vi "AeroFlowSanitiser.vi"(9 "Error_Flags":dbl[](array[numeric])=[200000.0, 200000.0, 200000.0, 200000.0, 200001.0, 200000.0, 200001.0, 200000.0, 200001.0, 200000.0, 200000.0, 200000.0, 200000.0, 200001.0, 200000.0, 200001.0, 200000.0, 200001.0, 200000.0, 200000.0, 200001.0, 200001.0, 200001.0, 200000.0, 200001.0, 200000.0, 200001.0, 200000.0, 200001.0, 200001.0, 200000.0, 200001.0, 200001.0, 200001.0, 200000.0, 200001.0, 200000.0, 200000.0, 200000.0, 200001.0, 200001.0, 200001.0, 200000.0, 200000.0, 200000.0, 200000.0, 200000.0, 200000.0, 200001.0, 200000.0, 200001.0, 200001.0, 200001.0, 200000.0, 200001.0, 200000.0, 200000.0, 200000.0, 200000.0, 200001.0, 200000.0, 200001.0, 200000.0, 200001.0, 200001.0, 200001.0, 200001.0, 200001.0, 200001.0, 200001.0, 200001.0, 200001.0, 200001.0, 200001.0, 200001.0, 200001.0, 200001.0, 200001.0, 200000.0, 200001.0, 200001.0, 200001.0, 200001.0, 200001.0, 200000.0, 200000.0, 200001.0, 200000.0, 200000.0, 200000.0, 200001.0, 200001.0, 200000.0, 200001.0, 200000.0, 200000.0, 200000.0, 200000.0, 200000.0, 200000.0, 200000.0, 200001.0, 200000.0, 200001.0, 200000.0, 200000.0, 200000.0, 200000.0, 200000.0, 200000.0, 200000.0, 200000.0, 200000.0, 200000.0, 200000.0, 200001.0, 200001.0, 200001.0, 200000.0, 200000.0, 200000.0, 200000.0, 200001.0, 200000.0, 200000.0, 200000.0, 200001.0, 200001.0, 200000.0, 200000.0, 200000.0, 200001.0, 200000.0, 200000.0, 200001.0, 200000.0, 200001.0, 200001.0, 200001.0, 200000.0, 200001.0, 200001.0, 200001.0, 200001.0, 200001.0, 200001.0, 200001.0, 200001.0, 200001.0, 200001.0, 200001.0, 200001.0, 200001.0, 200000.0, 200000.0, 200000.0, 200000.0, 200000.0, 200001.0, 200001.0, 200001.0, 200001.0, 200001.0, 200001.0, 200001.0, 200001.0, 200001.0, 200001.0, 200001.0, 200000.0, 200001.0, 200001.0, 200001.0, 200001.0, 200001.0, 200001.0, 200000.0, 200001.0, 200001.0, 200001.0, 200001.0, 200001.0, 200001.0, 200000.0, 200001.0, 200001.0, 200001.0, 200000.0, 200001.0, 200000.0, 200000.0, 200001.0, 200001.0, 200001.0, 200001.0, 200001.0, 200001.0, 200000.0, 200000.0, 200000.0, 200001.0, 200001.0, 200001.0, 200001.0, 200000.0, 200001.0, 200001.0, 200001.0, 200001.0, 200000.0, 200001.0, 200001.0, 200001.0, 200001.0, 200000.0, 200001.0, 200000.0, 200001.0, 200001.0, 200001.0, 200001.0, 200001.0, 200001.0, 200001.0, 200001.0, 200001.0, 200001.0, 200001.0, 200001.0, 200001.0, 200001.0, 200001.0, 200001.0, 200001.0, 200000.0, 200001.0, 200001.0, 200001.0, 200001.0, 200001.0, 200000.0, 200001.0, 200001.0, 200001.0, 200000.0, 200000.0, 200001.0, 200000.0, 200001.0, 200001.0, 200001.0, 200001.0, 200001.0, 200001.0, 200001.0, 200001.0, 200001.0, 200001.0, 200001.0, 200001.0, 200000.0, 200001.0, 200001.0, 200000.0, 200001.0, 200000.0, 200001.0, 200000.0, 200001.0, 200001.0, 200001.0, 200001.0, 200001.0, 200001.0, 200001.0, 200000.0, 200001.0, 200001.0, 200000.0, 200001.0, 200001.0, 200001.0, 200001.0, 200001.0, 200000.0, 200001.0, 200001.0, 200001.0, 200000.0, 200001.0, 200000.0, 200000.0, 200001.0, 200001.0, 200001.0, 200000.0, 200001.0, 200000.0, 200001.0, 200000.0, 200000.0, 200000.0, 200000.0, 200000.0, 200000.0, 200001.0, 200000.0, 200000.0, 200000.0, 200000.0, 200000.0, 200001.0, 200000.0, 200000.0, 200001.0, 200001.0, 200001.0, 200000.0, 200000.0, 200100.0, 200000.0, 200001.0, 200001.0, 200001.0, 200000.0, 200001.0, 200001.0, 200001.0, 200000.0, 200001.0, 200000.0, 200001.0, 200000.0, 200000.0, 200000.0, 200000.0, 200000.0, 200000.0, 200000.0, 200000.0, 200001.0, 200001.0, 200001.0, 200001.0, 200000.0, 200001.0, 200001.0, 200001.0, 200001.0, 200001.0, 200001.0, 200001.0, 200001.0, 200001.0, 200001.0, 200001.0, 200001.0, 200001.0, 200000.0, 200000.0, 200001.0, 200000.0, 200000.0, 200001.0, 200001.0, 200001.0, 200000.0, 200001.0, 200000.0, 200000.0, 200001.0, 200000.0, 200000.0, 200001.0, 200001.0, 200000.0, 200001.0, 200001.0, 200100.0, 200001.0, 200001.0, 200001.0, 200001.0, 200000.0, 200001.0, 200000.0, 200001.0, 200001.0, 200001.0, 200001.0, 200001.0, 200001.0, 200000.0, 200001.0, 200000.0, 200001.0, 200001.0, 200001.0, 200000.0, 200001.0, 200000.0, 200001.0, 200000.0, 200000.0, 200001.0, 200001.0, 200001.0, 200001.0, 200001.0, 200001.0, 200000.0, 200000.0, 200001.0, 200001.0, 200001.0, 200001.0, 200000.0, 200001.0, 200000.0, 200001.0, 200001.0, 200001.0, 200001.0, 200001.0, 200001.0, 200001.0, 200001.0, 200001.0, 200001.0, 200001.0, 200001.0, 200001.0, 200001.0, 200001.0, 200001.0, 200001.0, 200000.0, 200000.0, 200000.0, 200000.0, 200000.0, 200000.0, 200001.0, 200001.0, 200000.0, 200001.0, 200000.0, 200001.0, 200001.0, 200001.0, 200000.0, 200001.0, 200000.0, 200001.0, 200001.0, 200000.0, 200001.0, 200000.0, 200001.0, 200001.0, 200000.0, 200100.0, 200001.0, 200001.0, 200000.0, 200001.0, 200001.0, 200001.0, 200001.0, 200001.0, 200001.0, 200001.0, 200000.0, 200001.0, 200000.0, 200000.0, 200001.0, 200001.0, 200001.0, 200001.0, 200001.0, 200001.0, 200001.0, 200001.0, 200001.0, 200001.0, 200001.0, 200001.0, 200001.0, 200001.0, 200001.0, 200001.0, 200001.0, 200100.0, 200000.0, 200001.0, 200001.0, 200001.0, 200001.0, 200000.0, 200001.0, 200001.0, 200001.0, 200000.0, 200001.0, 200000.0, 200000.0, 200001.0, 200001.0, 200000.0, 200000.0, 200001.0, 200001.0, 200001.0, 200001.0, 200001.0, 200001.0, 200001.0, 200001.0, 200000.0, 200000.0, 200001.0, 200001.0, 200000.0, 200001.0, 200001.0, 200001.0, 200001.0, 200001.0, 200001.0, 200001.0, 200001.0, 200001.0, 200001.0, 200001.0, 200001.0, 200001.0, 200001.0, 200001.0, 200001.0, 200000.0, 200000.0, 200000.0, 200000.0, 200000.0, 200001.0, 200000.0, 200001.0, 200001.0, 200001.0, 200001.0, 200001.0, 200001.0, 200001.0, 200000.0, 200000.0, 200000.0, 200001.0, 200001.0, 200000.0, 200001.0, 200000.0, 200001.0, 200001.0, 200001.0, 200000.0, 200000.0, 200001.0, 200001.0, 200001.0, 200001.0, 200001.0, 200001.0, 200001.0, 200000.0, 200001.0, 200000.0, 200001.0, 200001.0, 200000.0, 200001.0, 200000.0, 200001.0, 200001.0, 200001.0, 200001.0, 200001.0, 200001.0, 200001.0, 200001.0, 200000.0, 200001.0, 200000.0, 200001.0, 200000.0, 200000.0, 200000.0, 200000.0, 200000.0, 200000.0, 200000.0, 200000.0, 200000.0, 200000.0, 200001.0, 200001.0, 200000.0, 200001.0, 200000.0, 200001.0, 200000.0, 200000.0, 200000.0, 200000.0, 200001.0, 200000.0, 200000.0, 200001.0, 200001.0, 200001.0, 200000.0, 200000.0, 200000.0, 200000.0, 200000.0, 200000.0, 200000.0, 200000.0, 200000.0, 200000.0, 200000.0, 200000.0, 200000.0, 200000.0, 200001.0, 200000.0, 200000.0, 200000.0, 200001.0, 200000.0, 200000.0, 200000.0, 200001.0, 200001.0, 200001.0, 200001.0, 200001.0, 200001.0, 200001.0, 200000.0, 200000.0, 200001.0, 200001.0, 200001.0, 200001.0, 200001.0, 200001.0, 200001.0, 200001.0, 200001.0, 200000.0, 200001.0, 200001.0, 200001.0, 200001.0, 200001.0, 200000.0, 200001.0, 200000.0, 200000.0, 200001.0, 200001.0, 200001.0, 200001.0, 200001.0, 200000.0, 200001.0, 200000.0, 200001.0, 200001.0, 200001.0, 200001.0, 200000.0, 200001.0, 200001.0, 200000.0, 200001.0, 200001.0, 200001.0, 200001.0, 200001.0, 200001.0, 200001.0, 200001.0, 200001.0, 200001.0, 200000.0, 200001.0, 200000.0, 200001.0, 200001.0, 200000.0, 200000.0, 200000.0, 200000.0, 200000.0, 200001.0, 200001.0, 200001.0, 200000.0, 200001.0, 200000.0, 200000.0, 200001.0, 200001.0, 200001.0, 200001.0, 200001.0, 200001.0, 200001.0, 200000.0, 200001.0, 200000.0, 200001.0, 200001.0, 200001.0, 200001.0, 200001.0, 200001.0, 200001.0, 200001.0, 200000.0, 200000.0, 200001.0, 200001.0, 200001.0, 200001.0, 200001.0, 200001.0, 200001.0, 200001.0, 200001.0, 200000.0, 200001.0, 200001.0, 200001.0, 200001.0, 200001.0, 200001.0, 200001.0, 200001.0, 200001.0, 200001.0, 200001.0, 200001.0, 200000.0, 200001.0, 200000.0, 200001.0, 200001.0, 200001.0, 200001.0, 200001.0, 200001.0, 200001.0, 200001.0, 200100.0, 200000.0, 200001.0, 200000.0, 200000.0, 200001.0, 200001.0, 200001.0, 200001.0, 200001.0, 200001.0, 200001.0, 200001.0, 200001.0, 200001.0, 200001.0, 200001.0, 200000.0, 200000.0, 200001.0, 200001.0, 200001.0, 200001.0, 200001.0, 200001.0, 200001.0, 200001.0, 200001.0, 200001.0, 200001.0, 200000.0, 200001.0, 200001.0, 200001.0, 200000.0, 200001.0, 200000.0, 200001.0, 200001.0, 200000.0, 200001.0, 200000.0, 200001.0, 200001.0, 200001.0, 200001.0, 200000.0, 200001.0, 200000.0, 200001.0, 200000.0, 200001.0, 200001.0, 200000.0], 11 "VmagUVWConeDirty":dbl[][](array[numeric])=array820x5[4100 elements]) -> (1 "GoodFraction":dbl, 3 "VmagUVWConeClean":dbl[][](array[numeric]))   [LabVIEW 2013]
panel:
  out "TotalPoints":i32
  out "ValidPoints":i32
  out "InvalidPoints":i32
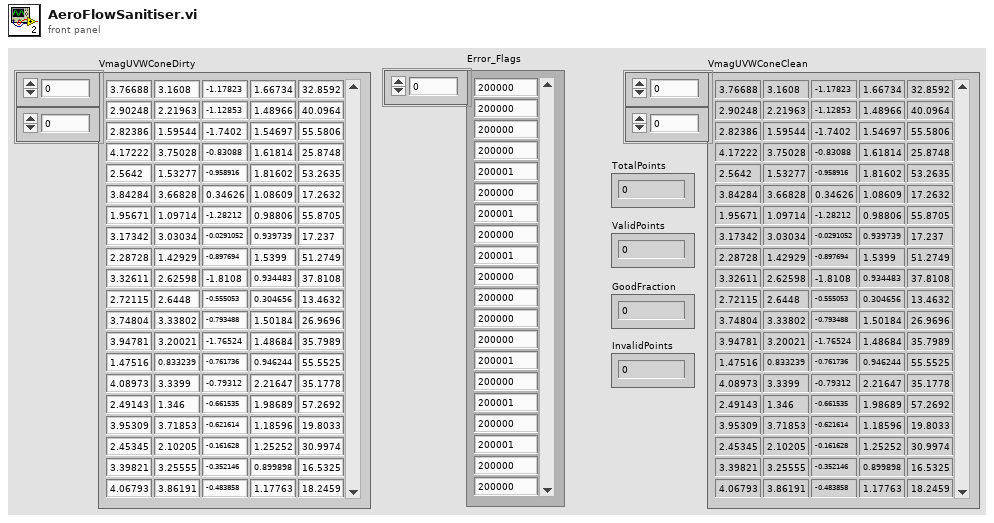
[diagram p1: front panel]
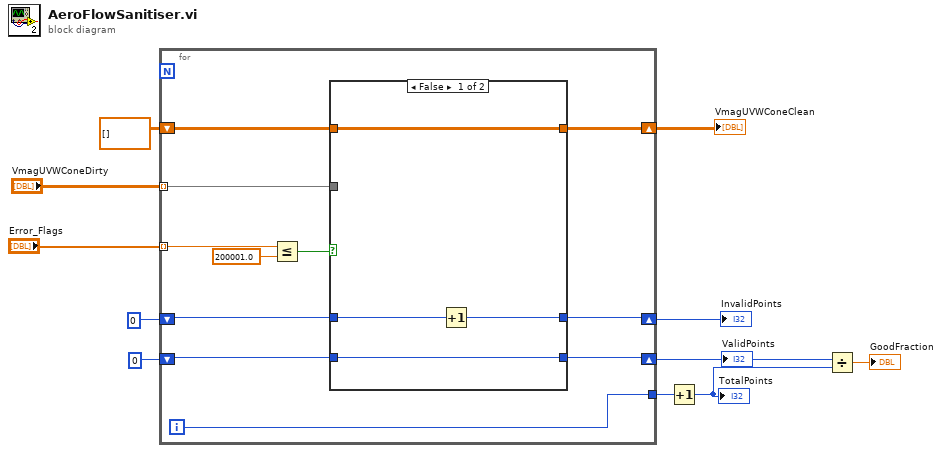
[diagram p0: block diagram]
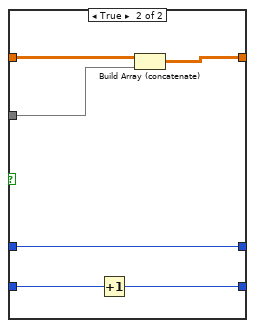
[diagram p2: hidden frame]
diagram:
  n1 = for {
    tunnel: "VmagUVWConeDirty" -> [w19] mode=indexing
    tunnel: "Error_Flags" -> [w22] mode=indexing
    shift-right: [w17] -> w8
    shift-left: dbl[][] [] -> [w18]
    shift-right: [w15] -> w4
    shift-left: 0 -> [w16]
    shift-right: [w14] -> w3
    shift-left: 0 -> [w13]
    tunnel: [w12] -> w5
    i -> [w12]
    n2 = Less Or Equal?(x=w22, y=200001.0) -> (x <= y?=w20:bool)
    n3 = case shown="False" w20 {
      tunnel: w19 -> [_ w32]
      tunnel: w18 -> [w26 w31]
      tunnel: [w26 w30] -> w17
      tunnel: w16 -> [w25 w29]
      tunnel: [w24 w29] -> w15
      tunnel: w13 -> [w23 w28]
      tunnel: [w23 w27] -> w14
      frame False {
        n4 = Increment(x=w25) -> (x+1=w24:i32)
      }
      frame True {
        n5 = Increment(x=w28) -> (x+1=w27:i32)
        n6 = Build Array (concatenate)(w31, w32) -> (w30:dbl[][])
      }
    }
  }
  "VmagUVWConeClean" <- w8
  "InvalidPoints" <- w4
  "ValidPoints" <- w3
  n7 = Increment(x=w5) -> (x+1=w2:i32)
  "TotalPoints" <- w2
  n8 = Divide(x=w3, y=w2) -> (x/y=→"GoodFraction":dbl)
